vi "Move DC_2_Distance.vi"(0 "NXT":T3, 1 "DC Motors":T2={"DC Motor"=enum."DC Motor", "Address"=-1, "Address"=-1}, 2 "Return Mode (When Move Completes)":u16(ring) items=["When Move Completes", "Immediately"], 3 "Timeout (2.5 sec)":sgl=2.5, 5 "Encoder Counts 1":i32=100, 7 "Speed 1 (100)":i8=100, 9 "Encoder Counts 2":i32=100, 11 "Speed 2 (100)":i8=100) -> (4 "NXT":T3)   [LabVIEW 2012, in "4134Outputs.lvlib"]
uses:
  4134Outputs.lvlib
  <vilib>/NXT/Subs/LVHSConnector.ctl
  <vilib>/NXT/LegoClasses/BrickReference/BrickReference.lvclass
  <vilib>/NXT/Subs/MotorXNode.DC Motor Type.ctl
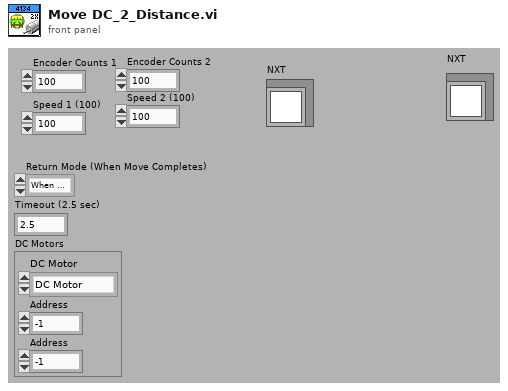
[diagram p1: front panel]
types:
  T1 = typedef "MotorXNode.DC Motor Type.ctl" = enum16{"DC Motor"}
  T2 = cluster{"DC Motor":T1, "Address":i16, "Address":i16}
  T3 = typedef "LVHSConnector.ctl" = refnum<class "BrickReference.lvclass">
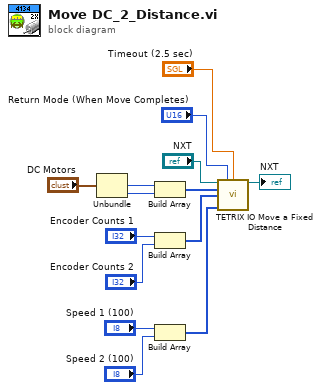
[diagram p0: block diagram]
diagram:
  n1 = Unbundle("DC Motors") -> ("Address"=w14:i16, "Address"=w3:i16)  [unwired: 1 out]
  n2 = Build Array(w14, w3) -> (w5:i16[])
  n3 = Build Array("Encoder Counts 1", "Encoder Counts 2") -> (w9:i32[])
  n4 = Build Array("Speed 1 (100)", "Speed 2 (100)") -> (w8:i8[])
  n5 = call <vilib>:"TETRIX IO Move a Fixed Distance.vi"("NXT"="NXT", "VI Returns (When Move Completes)"="Return Mode (When Move Completes)", "Timeout (2.5 sec)"="Timeout (2.5 sec)", "DC Motors"=w5, "Encoder Counts"=w9, "Speed (0)"=w8) -> ("NXT"=→"NXT":T3)  [unwired: 9 in]
